vi "ChangeConfirm.vi"(0 "Data input":T1, 5 "error in":errorcluster) -> (14 "Data ouput":T1, 19 "error out":errorcluster)   [LabVIEW 2018]
doc: "<B>This VI is used for setting a new value to the selected property.</B>"
uses:
  Ctrl/Data.ctl
  Ctrl/Caps.ctl
  Ctrl/Property.ctl
  Ctrl/PhysicalChannel.ctl
  Ctrl/Register.ctl
  Ctrl/Bitfield.ctl
  Ctrl/Scale.ctl
  Ctrl/ScaleType.ctl
  Ctrl/Enum.ctl
  Ctrl/EnumValue.ctl
  Ctrl/compond commands.ctl
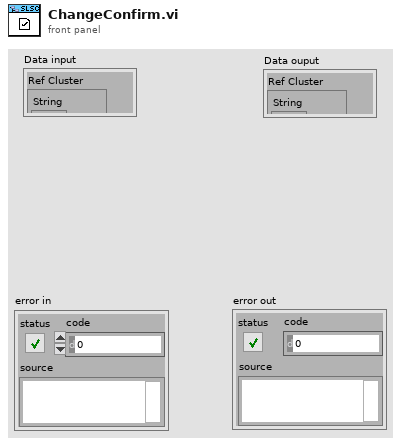
[diagram p1: front panel]
types:
  T1 = typedef "Data.ctl" = cluster{"Ref Cluster":cluster{"String":refnum<vi>, "U8":refnum<vi>, "I8":refnum<vi>, "U32":refnum<vi>, "I32":refnum<vi>, "U64":refnum<vi>, "I64":refnum<vi>, "Ring":refnum<vi>, "DBL":refnum<vi>, "Add":refnum<vi>, "Remove":refnum<vi>, "Property tree":refnum<vi>, "confirm":refnum<vi>}, "JSON Text":string, "Original JSON Text":string, "Caps":T2, "SLSC Output Tree":cluster{"Left Cell String":string, "Child Text":string[], "Child Tag":string, "Item Indent":i32, "Child Only?":bool, "Glyph Index":i32, "offline value":variant}[], "Ref Index and Control Type":cluster{"index":i32, "Datatype":string}, "Selected Type and name":cluster{"Selected Type":enum16{"Property", "Physical Channel", "Other"}, "Selected Property Name":string}, "Update whole Tree?":bool}
  T2 = typedef "Caps.ctl" = cluster{"properties":T3[], "physical channels":T4[], "registers":T5[], "scales":T7[], "enums":T9[], "productName":string}
  T3 = typedef "Property.ctl" = cluster{"name":string, "bitfield":string, "value":variant, "dataType":string, "min":variant, "max":variant, "scale":string, "access":string}
  T4 = typedef "PhysicalChannel.ctl" = cluster{"name":string, "properties":T3[]}
  T5 = typedef "Register.ctl" = cluster{"name":string, "address":i32, "size":i32, "bitfields":T6[], "initialValue":variant, "connectedProperties":string[]}
  T6 = typedef "Bitfield.ctl" = cluster{"name":string, "offset":i32, "size":i32, "signed":bool}
  T7 = typedef "Scale.ctl" = cluster{"name":string, "type":T8, "params":variant}
  T8 = typedef "ScaleType.ctl" = enum16{"NoScale", "Table", "Polynomial", "Linear"}
  T9 = typedef "Enum.ctl" = cluster{"name":string, "values":T10[]}
  T10 = typedef "EnumValue.ctl" = cluster{"name":string, "value":i32}
  T11 = typedef "compond commands.ctl" = enum16{"Get Property Array", "Get Physical Channel Property Array", "Get the Selected Position", "Get Property and Physical Channel Name", "Get Type and Value", "Make and Set a new Property", "Modify the Value", "Delete a Property"}
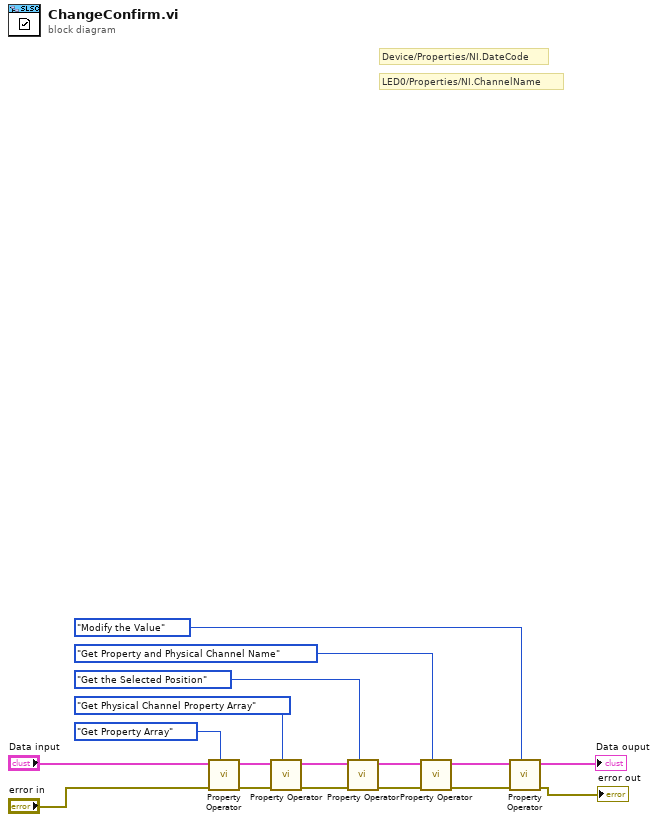
[diagram p0: block diagram]
diagram:
  # "LED0/Properties/NI.ChannelName"
  # "Device/Properties/NI.DateCode"
  n1 = call "Property Operator.vi"("Command"=compond_commands."Get Property Array", "error in"="error in", "Data"="Data input") -> ("error out"=w13:errorcluster, "Data 2"=w14:T1)  [unwired: 6 in, 1 out]
  n2 = call "Property Operator.vi"("Command"=compond_commands."Get Physical Channel Property Array", "error in"=w13, "Data"=w14) -> ("error out"=w11:errorcluster, "Data 2"=w12:T1)  [unwired: 6 in, 1 out]
  n3 = call "Property Operator.vi"("Command"=compond_commands."Get the Selected Position", "error in"=w11, "Data"=w12) -> ("error out"=w7:errorcluster, "Data 2"=w8:T1)  [unwired: 6 in, 1 out]
  n4 = call "Property Operator.vi"("Command"=compond_commands."Get Property and Physical Channel Name", "error in"=w7, "Data"=w8) -> ("error out"=w5:errorcluster, "Data 2"=w6:T1)  [unwired: 6 in, 1 out]
  n5 = call "Property Operator.vi"("Command"=compond_commands."Modify the Value", "error in"=w5, "Data"=w6) -> ("error out"=→"error out":errorcluster, "Data 2"=→"Data ouput":T1)  [unwired: 6 in, 1 out]
